vi "tm.vi"(8 "change":bool, 10 "输入簇":T2(array[cluster]), 11 "apply":bool) -> (2 "输出簇":T2(array[cluster]))   [LabVIEW 2018]
panel:
  in  "8":T1
  in  "7":T1
  in  "6":T1
  in  "5":T1
  in  "4":T3
  in  "3":T3
  in  "2":T3
  in  "1":T1
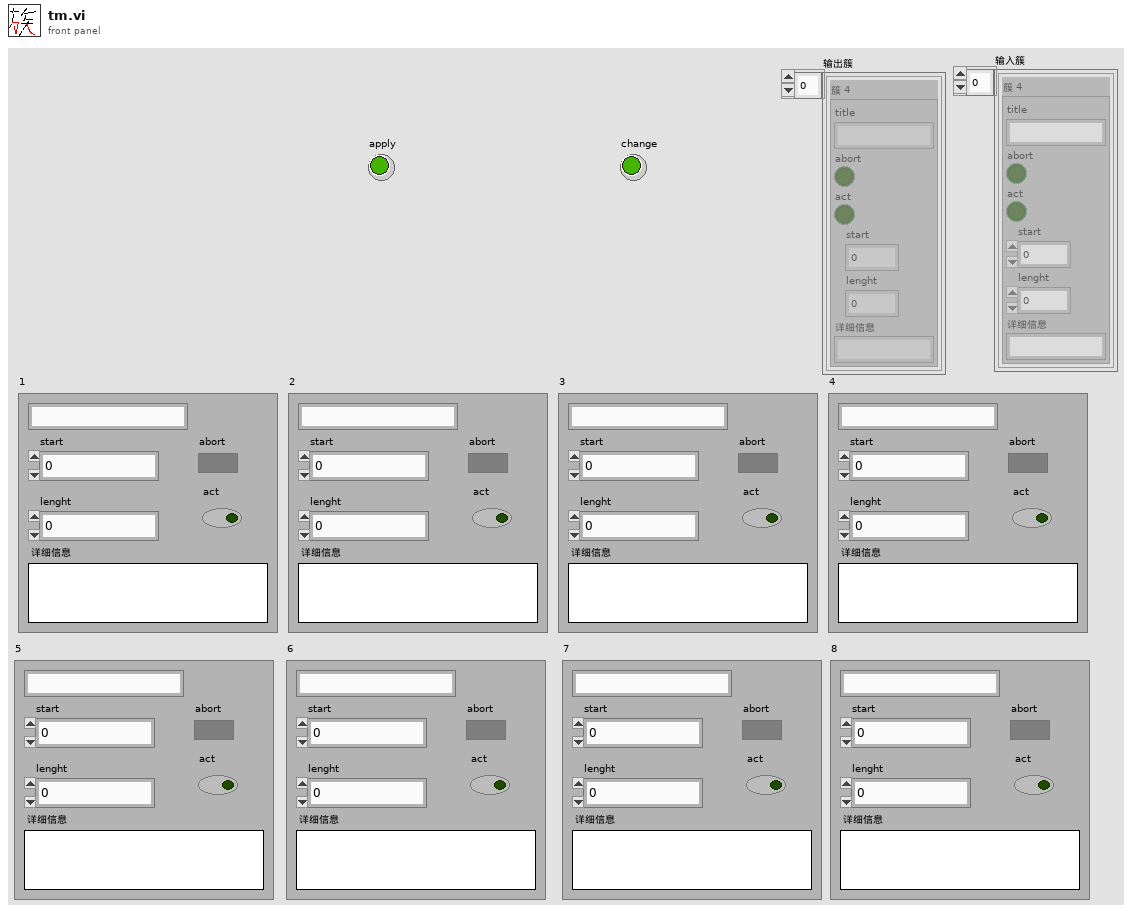
[diagram p1: front panel]
types:
  T1 = cluster{"title\ntitle":string, "abort":bool, "act":bool, "start":dbl, "lenght":dbl, "详细信息":string}
  T2 = cluster{"簇 4":cluster{"title":string, "abort":bool, "act":bool, "start":dbl, "lenght":dbl, "详细信息":string}}[]
  T3 = cluster{"title":string, "abort":bool, "act":bool, "start":dbl, "lenght":dbl, "详细信息":string}
  T4 = cluster{"8":cluster{"title\ntitle":string, "abort":bool, "act":bool, "start":dbl, "lenght":dbl, "详细信息":string}}[]
  T5 = cluster{"簇 4":cluster{"title":string, "abort":bool, "act":bool, "start":dbl, "lenght":dbl, "详细信息":string}}
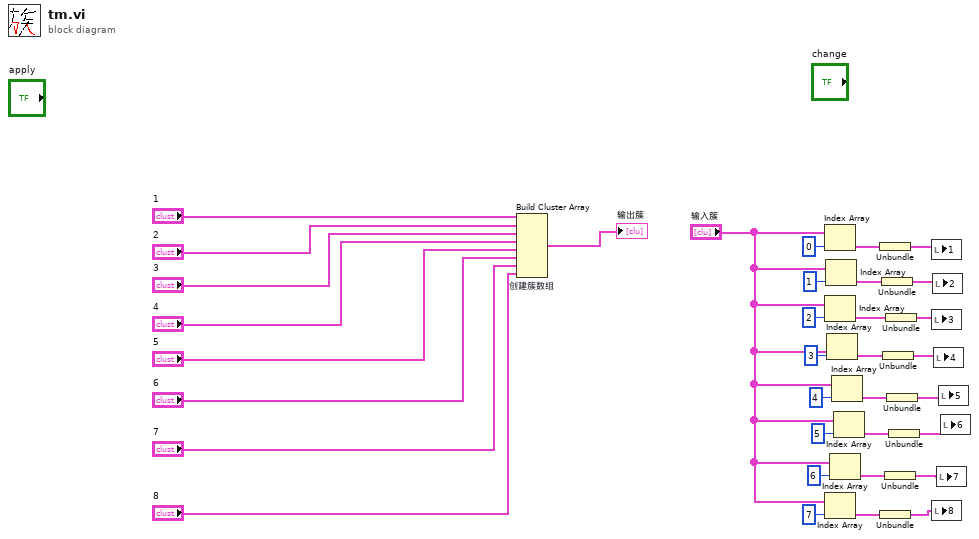
[diagram p0: block diagram]
diagram:
  n1 = Build Cluster Array "创建簇数组"("1", "2", "3", "4", "5", "6", "7", "8") -> (→"输出簇":T4)
  n2 = Index Array(array="输入簇", index=0 ("索引")) -> (element=w29:T5)
  n3 = Index Array(array="输入簇", index=2 ("索引")) -> (element=w23:T5)
  n4 = Index Array(array="输入簇", index=7 ("索引")) -> (element=w6:T5)
  n5 = Index Array(array="输入簇", index=1 ("索引")) -> (element=w24:T5)
  n6 = Index Array(array="输入簇", index=3 ("索引")) -> (element=w18:T5)
  n7 = Index Array(array="输入簇", index=6 ("索引")) -> (element=w9:T5)
  n8 = Index Array(array="输入簇", index=4 ("索引")) -> (element=w13:T5)
  n9 = Index Array(array="输入簇", index=5 ("索引")) -> (element=w10:T5)
  n10 = Unbundle(w29) -> ("簇 4"=w28:T3)
  n11 = Unbundle(w6) -> ("簇 4"=w1:T3)
  n12 = Unbundle(w24) -> ("簇 4"=w25:T3)
  n13 = Unbundle(w18) -> ("簇 4"=w19:T3)
  n14 = Unbundle(w9) -> ("簇 4"=w2:T3)
  n15 = Unbundle(w23) -> ("簇 4"=w22:T3)
  n16 = Unbundle(w13) -> ("簇 4"=w4:T3)
  n17 = Unbundle(w10) -> ("簇 4"=w3:T3)
  n18 = local write "1"(w28) -> ()
  n19 = local write "3"(w22) -> ()
  n20 = local write "8"(w1) -> ()
  n21 = local write "2"(w25) -> ()
  n22 = local write "4"(w19) -> ()
  n23 = local write "7"(w2) -> ()
  n24 = local write "5"(w4) -> ()
  n25 = local write "6"(w3) -> ()
